vi "Read Frame Rate.vi"(8 "error in (no error)":errorcluster, 11 "Camera Simulator in":refnum<class "Camera Simulator.lvclass">) -> (0 "error out":errorcluster, 2 "Frame Rate":u32, 3 "Camera Simulator out":refnum<class "Camera Simulator.lvclass">)   [LabVIEW 2020, in "Camera Simulator.lvlib" / "Camera Simulator.lvclass"]
uses:
  Camera Simulator.lvclass
  Camera Simulator.lvclass/Camera Simulator.ctl
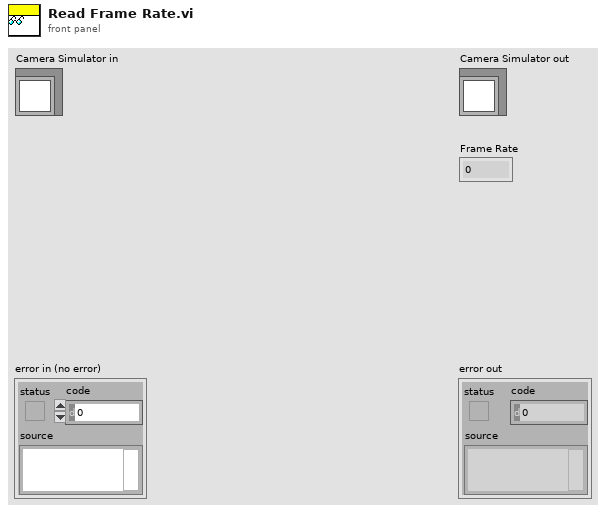
[diagram p1: front panel]
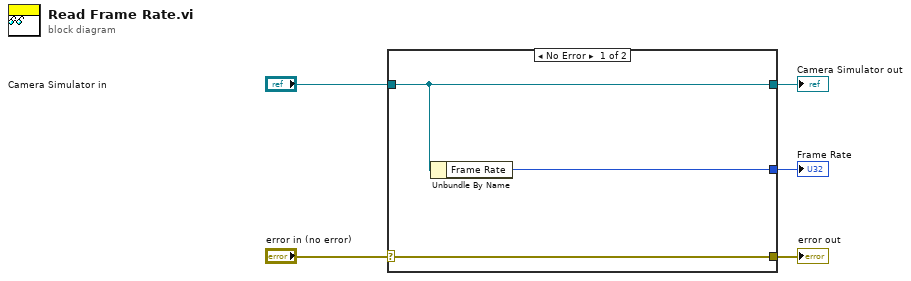
[diagram p0: block diagram]
diagram:
  n1 = case shown="No Error" "error in (no error)" {
    selector: "error in (no error)" -> [w8 w9]
    tunnel: [w8 w9] -> w4
    tunnel: [w7 w10] -> w2
    tunnel: "Camera Simulator in" -> [w7 w10]
    tunnel: [w6 _] -> w1
    frame No Error {
      n2 = Unbundle By Name(w7) -> ("Frame Rate"=w6:u32)
    }
    frame Error {
    }
  }
  "error out" <- w4
  "Camera Simulator out" <- w2
  "Frame Rate" <- w1
